vi "GetSourceName.vi"(6 "error in":errorcluster, 9 "Terminal in":refnum<class "Terminal.lvclass">) -> (0 "error out":errorcluster, 3 "Terminal out":refnum<class "Terminal.lvclass">, 4 "source":string)   [LabVIEW 2014, in "Raspberry Pi Compatible Compiler for LabVIEW.lvlib" / "Terminal.lvclass"]
uses:
  Terminal.lvclass
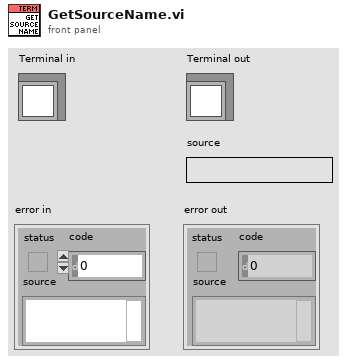
[diagram p1: front panel]
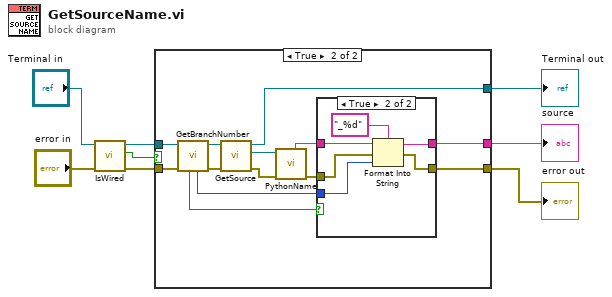
[diagram p0: block diagram]
diagram:
  n1 = call "IsWired.vi"("error in"="error in", "Terminal in"="Terminal in") -> ("error out"=w2:errorcluster, "wired"=w1:bool, "Terminal out"=w3:refnum<class "Terminal.lvclass">)  [unwired: 5 in]
  n2 = case shown="True" w1 {
    tunnel: [_ w17] -> w8
    tunnel: [w10 w16] -> w7
    tunnel: [w9 w13] -> w6
    tunnel: w3 -> [w10 w12]
    tunnel: w2 -> [w9 w11]
    frame False {
    }
    frame True {
      n3 = call "GetBranchNumber.vi"("error in"=w11, "Terminal in"=w12) -> ("error out"=w19:errorcluster, "Terminal out"=w20:refnum<class "Terminal.lvclass">, "branch"=w15:i32, "wire branched"=w21:bool)  [unwired: 4 in]
      n4 = call "GetSource.vi"("error in"=w19, "Terminal in"=w20) -> ("error out"=w22:errorcluster, "source"=w23:refnum<class "Terminal.lvclass">, "Terminal out"=w16:refnum<class "Terminal.lvclass">)  [unwired: 5 in]
      n5 = call-dynamic "PythonName.vi"("error in"=w22, "Terminal in"=w23) -> ("error out"=w14:errorcluster, "name"=w18:string)  [unwired: 6 in, 2 out]
      n6 = case shown="True" w21 {
        tunnel: w18 -> [w25 w31]
        tunnel: [w25 w30] -> w17
        tunnel: w15 -> [_ w28]
        tunnel: w14 -> [w24 w26]
        tunnel: [w24 w27] -> w13
        frame False {
        }
        frame True {
          n7 = Format Into String(format string="_%d", initial string=w31, error in=w26, w28) -> (resulting string=w30:string, error out=w27:errorcluster)
        }
      }
    }
  }
  "error out" <- w6
  "Terminal out" <- w7
  "source" <- w8
